vi "Report Gen Title_Folder.vi"() -> ()   [LabVIEW 2021]
uses:
  <vilib>/Utility/file.llb/Read Delimited Spreadsheet (string).vi
  <vilib>/Utility/file.llb/Write Delimited Spreadsheet (string).vi
panel:
  in  "appended array 2":string[][](array[string])
  in  "1D data":string[](array[string])
  out "output array":string[](array[string])
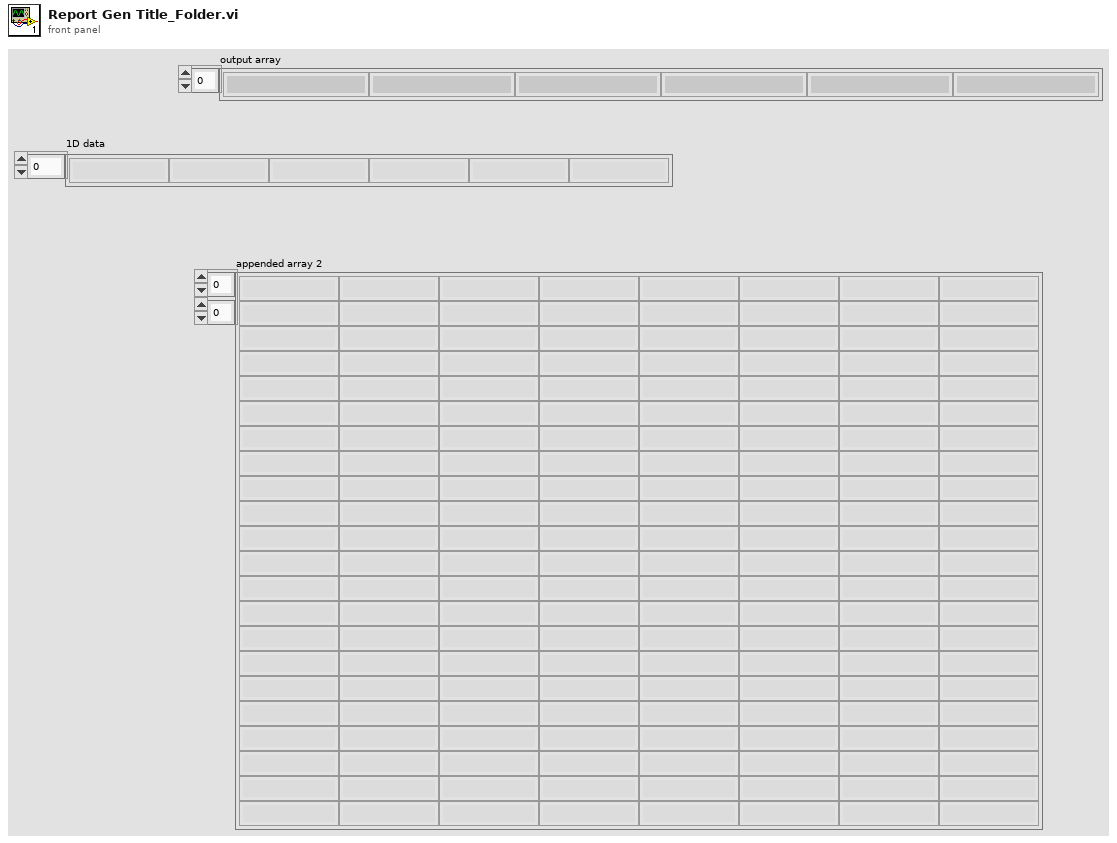
[diagram p1: front panel]
types:
  T1 = enum16{"open", "replace", "create", "open or create", "replace or create", "replace or create with confirmation"}
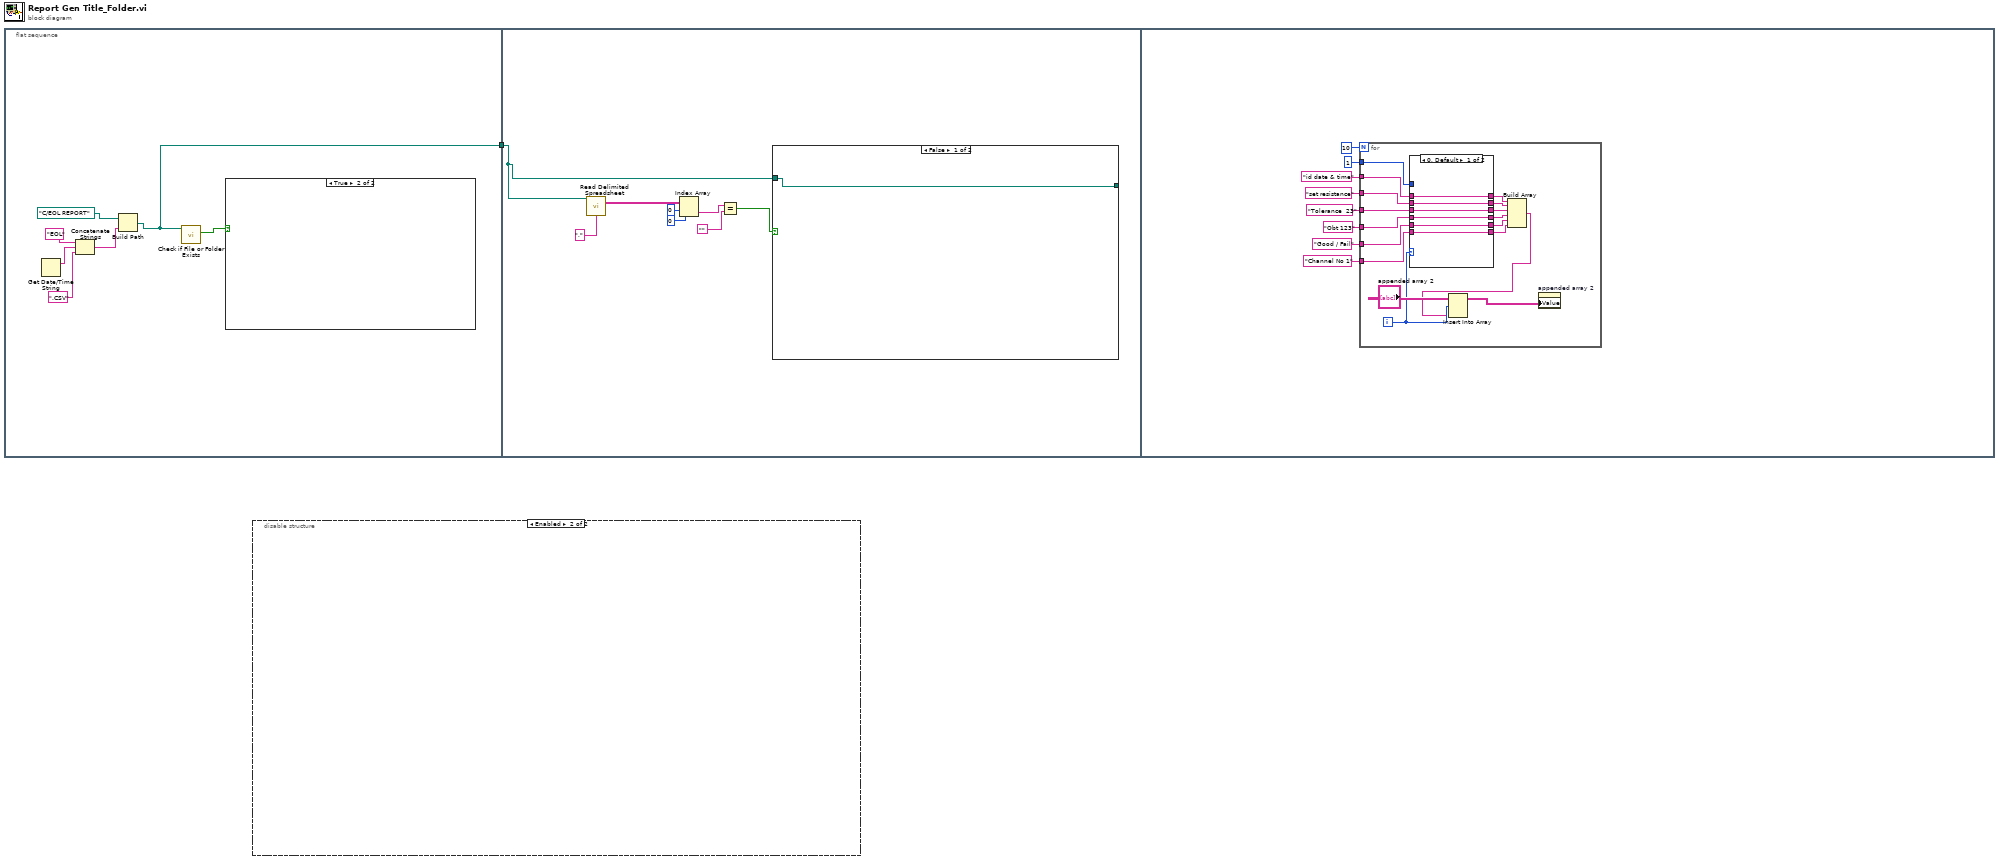
[diagram p0: block diagram]
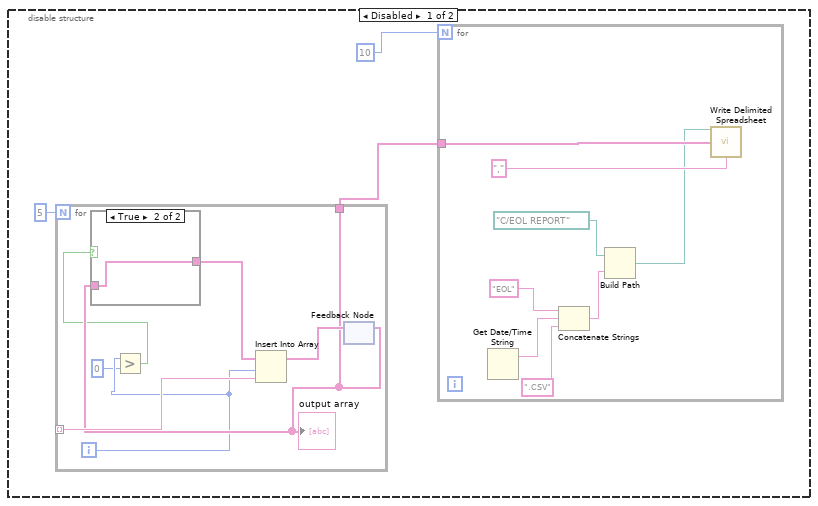
[diagram p2: hidden frame]
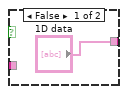
[diagram p3: hidden frame]
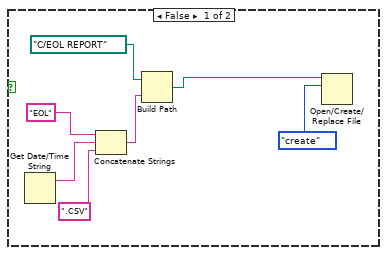
[diagram p4: hidden frame]
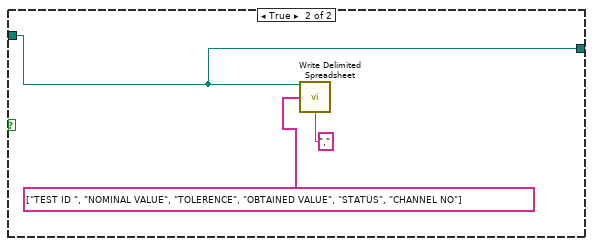
[diagram p5: hidden frame]
diagram:
  n1 = flat-sequence {
    tunnel: [w2] -> w1
    tunnel: w1 -> [w16]
    frame #0 {
      n2 = Get Date/Time String() -> (date string=w4:string)  [unwired: 3 in, 1 out]
      n3 = Concatenate Strings("EOL", w4, ".CSV") -> (w6:string)
      n4 = Build Path(base path=path "C:/EOL REPORT" ("path"), name or relative path=w6) -> (appended path=w2:path)
      n5 = call <vilib>:"Check if File or Folder Exists.vi"("path"=w2) -> ("file or folder exists?"=w8:bool)  [unwired: 8 in, 2 out]
      n6 = case shown="True" w8 {
        frame False {
          n7 = Get Date/Time String() -> (date string=w12:string)  [unwired: 3 in, 1 out]
          n8 = Concatenate Strings("EOL", w12, ".CSV" ("string")) -> (w11:string)
          n9 = Build Path(base path=path "C:/EOL REPORT" ("path"), name or relative path=w11) -> (appended path=w9:path)
          n10 = Open/Create/Replace File(file path (use dialog)=w9, operation (0:open)=T1."create") -> ()  [unwired: 4 in, 3 out]
        }
        frame True {
        }
      }
    }
    frame #1 {
      n11 = call-poly <vilib>:"Read Delimited Spreadsheet.vi"("file path (dialog if empty)"=w16, "delimiter (\\t)"="," ("delimiter (\\t)")) -> ("all rows"=w22:string[][])  [unwired: 8 in, 5 out]
      n12 = Index Array(array=w22, index (row)=0, index (col)=0 ("disabled index (col)")) -> (element=w19:string)
      n13 = Equal?(x=w19, y="") -> (x = y?=w17:bool)
      n14 = case shown="False" w17 {
        tunnel: w16 -> [w24 w25]
        tunnel: [w24 w25] -> _
        frame False {
        }
        frame True {
          n15 = call-poly <vilib>:"Write Delimited Spreadsheet.vi"("file path (dialog if empty)"=w25, "1D data"=string[] ["TEST ID ", "NOMINAL VALUE", "TOLERENCE", "OBTAINED VALUE", "STATUS", "CHANNEL NO"], "delimiter (\\t)"="," ("delimiter (\\t)")) -> ()  [unwired: 11 in, 2 out]
        }
      }
    }
    frame #2 {
      n16 = for {
        N: 10 -> [_]
        tunnel: 1 -> [w52]
        tunnel: "id date & time" -> [w51]
        tunnel: "set resistance" -> [w49]
        tunnel: "Tolerance  23" -> [w47]
        tunnel: "Obt 123" -> [w45]
        tunnel: "Good / Fail" -> [w42]
        tunnel: "Channel No 1" -> [w40]
        i -> [w38]
        n17 = case shown="0, Default" w38 {
          tunnel: w52 -> [_ w71]
          tunnel: w51 -> [w58 w69]
          tunnel: [w58 w70] -> w50
          tunnel: w49 -> [w57 w68]
          tunnel: [w57 w67] -> w48
          tunnel: w47 -> [w56 w66]
          tunnel: [w56 w65] -> w46
          tunnel: w45 -> [w55 w64]
          tunnel: [w55 w63] -> w44
          tunnel: [w54 w62] -> w43
          tunnel: w42 -> [w54 w61]
          tunnel: [w53 w60] -> w41
          tunnel: w40 -> [w53 w59]
          frame 0, Default {
          }
          frame 1 {
            n18 = case shown="1" w71 {
              tunnel: [_ w77] -> w70
              tunnel: w69 -> [_ w77]
              tunnel: w68 -> [_ w76]
              tunnel: [_ w76] -> w67
              tunnel: w66 -> [_ w75]
              tunnel: [_ w75] -> w65
              tunnel: w64 -> [_ w74]
              tunnel: [_ w74] -> w63
              tunnel: [_ w73] -> w62
              tunnel: w61 -> [_ w73]
              tunnel: [_ w72] -> w60
              tunnel: w59 -> [_ w72]
              frame 0, Default {
              }
              frame 1 {
              }
            }
          }
        }
        n19 = Build Array(w50, w48, w46, w44, w43, w41) -> (w36:string[])
        n20 = Insert Into Array(array="appended array 2", index (row)=w38, new element=w36) -> (w37:string[][])  [unwired: 1 in]
        n21 = property on="appended array 2" class="Arr (strict)"("Value"=w37) -> ()  [unwired: 2 in, 2 out]
      }
    }
  }
  n22 = disable-structure shown="Enabled" {
    frame Disabled {
      n23 = for {
        N: 5 -> [_]
        tunnel: [w84] -> w80
        tunnel: _ -> [w87] mode=indexing
        i -> [w82]
        n24 = Greater?(x=w82, y=0) -> (0:w83:bool)
        n25 = feedback #1() -> (w84:string[])  [unwired: 1 in]
        "output array" <- w84
        n26 = case shown="True" w83 {
          tunnel: ["1D data" w89] -> w86
          tunnel: w84 -> [_ w89]
          frame False {
          }
          frame True {
          }
        }
        n27 = Insert Into Array(array=w86, index=w82, new element=w87) -> (w85:string[])
        n28 = feedback-in #1(w85) -> ()
      }
      n29 = for {
        N: 10 -> [_]
        tunnel: w80 -> [w96]
        n30 = Get Date/Time String() -> (date string=w93:string)  [unwired: 3 in, 1 out]
        n31 = Concatenate Strings("EOL", w93, ".CSV" ("string")) -> (w92:string)
        n32 = Build Path(base path=path "C:/EOL REPORT" ("path"), name or relative path=w92) -> (appended path=w90:path)
        n33 = call-poly <vilib>:"Write Delimited Spreadsheet.vi"("file path (dialog if empty)"=w90, "1D data"=w96, "delimiter (\\t)"="," ("delimiter (\\t)")) -> ()  [unwired: 11 in, 2 out]
      }
    }
    frame Enabled {
    }
  }
